vi "Set Sel Exp Group.vi"(8 "error in (no error)":errorcluster, 9 "Exp Group":refnum<class "Experiments_group.lvclass">, 10 "Group #":i32=-1, 11 "Control-Client in":refnum<class "Control-Client.lvclass">) -> (0 "error out":errorcluster, 3 "Control-Client out":refnum<class "Control-Client.lvclass">)   [LabVIEW 2018, in "Control-Client.lvclass"]
uses:
  Control-Client.lvclass
  Experiments/Experiments_group.lvclass
  Control-Client.lvclass/Control-Client.ctl
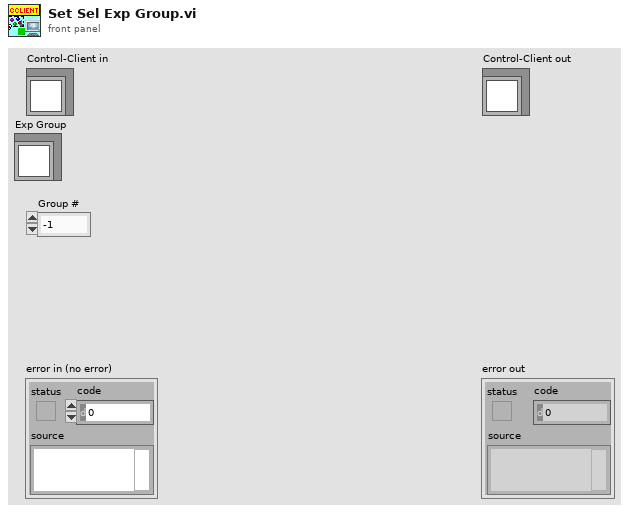
[diagram p1: front panel]
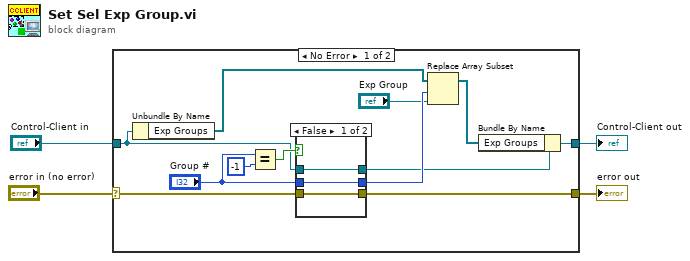
[diagram p0: block diagram]
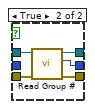
[diagram p2: hidden frame]
diagram:
  n1 = case shown="No Error" "error in (no error)" {
    selector: "error in (no error)" -> [w13 w25]
    tunnel: [w12 w25] -> w3
    tunnel: [w10 w26] -> w1
    tunnel: "Control-Client in" -> [w11 w26]
    frame No Error {
      n2 = Unbundle By Name(w11) -> ("Exp Groups"=w9:refnum<class "Experiments_group.lvclass">[])
      n3 = Equal?(x="Group #", y=-1) -> (x = y?=w15:bool)
      n4 = case shown="False" w15 {
        tunnel: [w19 w21] -> w8
        tunnel: "Group #" -> [w19 _]
        tunnel: w11 -> [w17 w24]
        tunnel: w13 -> [w18 w23]
        tunnel: [w18 w22] -> w12
        tunnel: [w17 w20] -> w5
        frame False {
        }
        frame True {
          n5 = call "Read Group #.vi"("error in (no error)"=w23, "Control-Client in"=w24) -> ("error out"=w22:errorcluster, "Group #"=w21:i32, "Control-Client out"=w20:refnum<class "Control-Client.lvclass">)  [unwired: 7 in]
        }
      }
      n6 = Replace Array Subset(array=w9, new element="Exp Group", index=w8) -> (w7:refnum<class "Experiments_group.lvclass">[])
      n7 = Bundle By Name(cluster=w5, "Exp Groups"=w7) -> (w10:refnum<class "Control-Client.lvclass">)
    }
    frame Error {
    }
  }
  "error out" <- w3
  "Control-Client out" <- w1
